vi "Find control by label.vi"(4 "error in":errorcluster, 6 "Control Label":string, 7 "Controls[]":refnum<vi>[](array[refnum])) -> (0 "error out":errorcluster, 1 "Found?":bool, 2 "Ctl Refnum":refnum<vi>, 3 "Controls[] dup":refnum<vi>[](array[refnum]))   [LabVIEW 2020]
doc: "Finds a control inside an array, that matches a label from an predefined enum listing valid controls."
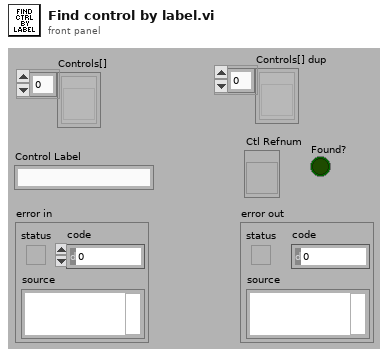
[diagram p1: front panel]
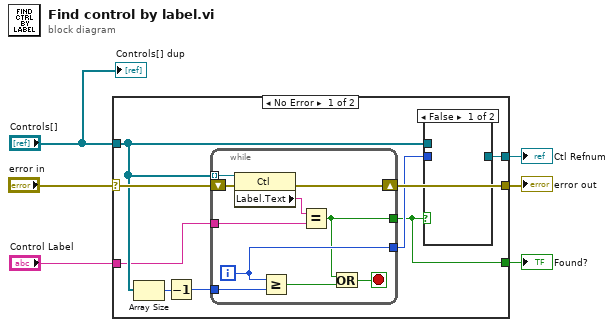
[diagram p0: block diagram]
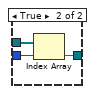
[diagram p2: hidden frame]
diagram:
  n1 = case shown="No Error" "error in" {
    selector: "error in" -> [w14 w29]
    tunnel: "Control Label" -> [w9 _]
    tunnel: "Controls[]" -> [w12 _]
    tunnel: [w15 w29] -> w5
    tunnel: [w13 _] -> w3
    tunnel: [w7 _] -> w1
    frame No Error {
      n2 = Array Size(array=w12) -> (size(s)=w11:i32)
      n3 = Decrement(x=w11) -> (x-1=w10:i32)
      n4 = while {
        tunnel: w12 -> [w28] mode=indexing
        shift-right: [w26] -> w15
        shift-left: w14 -> [w27]
        tunnel: w10 -> [w24]
        tunnel: w9 -> [w22]
        tunnel: [w20] -> w8
        tunnel: [w19] -> w7
        i -> [w20]
        stop <- w25 stop-if-true
        n5 = property class="Ctl"(reference=w28, error in=w27) -> (error out=w26:errorcluster, "Label.Text"=w21:string)  [unwired: 1 out]
        n6 = Greater Or Equal?(x=w20, y=w24) -> (x >= y?=w23:bool)
        n7 = Equal?(x=w21, y=w22) -> (x = y?=w19:bool)
        n8 = Or(x=w19, y=w23) -> (x .or. y?=w25:bool)
      }
      n9 = case shown="False" w7 {
        tunnel: [_ w18] -> w13
        tunnel: w12 -> [_ w17]
        tunnel: w8 -> [_ w16]
        frame False {
        }
        frame True {
          n10 = Index Array(array=w17, index=w16) -> (element=w18:refnum<vi>)
        }
      }
    }
    frame Error {
    }
  }
  "error out" <- w5
  "Ctl Refnum" <- w3
  "Found?" <- w1
  "Controls[] dup" <- "Controls[]"
